vi "Gui_Set_Lamp_Refs.vi"(8 "error in (no error)":errorcluster, 9 "Path":path, 10 "EXPERIMENT Inputs":T1={"Setup"="", "Date"="", "User Name"="", "Comment"="", "Experiment Procedures"=[], "Chemical Source"="", "Sample Components"=[], "Species"=[], "Laser 1"={"Used"=TRUE, "Name"="Spectroscopy", "Wavelength"=1000.0, "Energy"=25.0}, "Laser 2"={"Used"=TRUE, "Name"="Spectroscopy", "Wavelength"=1000.0, "Energy"=25.0}, "Laser 3"={"Used"=TRUE, "Name"="Spectroscopy", "Wavelength"=1000.0, "Energy"=25.0}, "Laser 4"={"Used"=TRUE, "Name"="Spectroscopy", "Wavelength"=1000.0, "Energy"=25.0}, "Laser 5"={"Used"=TRUE, "Name"="Spectroscopy", "Wavelength"=1000.0, "Energy"=25.0}, "Lamp 1"={"Used"=TRUE, "Name"="Spectroscopy", "Wavelength"=1000.0, "Attenuation"=25.0}, "Lamp 2"={"Used"=TRUE, "Name"="Spectroscopy", "Wavelength"=1000.0, "Attenuation"=25.0}, "Gas 1"={"Used"=TRUE, "Name"="Spectroscopy", "Pressure"=1000.0}, "Gas 2"={"Used"=TRUE, "Name"="Spectroscopy", "Pressure"=1000.0}, "Gas 3"={"Used"=TRUE, "Name"="Spectroscopy", "Pressure"=1000.0}, "Gas 4"={"Used"=TRUE, "Name"="Spectroscopy", "Pressure"=1000.0}, "Gas 5"={"Used"=TRUE, "Name"="Spectroscopy", "Pressure"=1000.0}}, 11 "Lamp Refs":refnum<vi>[](array[refnum])) -> (0 "error out":errorcluster caption="sortie d'erreur", 3 "Lamp Refs out":refnum<vi>[](array[refnum]))   [LabVIEW 2017]
uses:
  controls/EXPERIMENT_Inputs.ctl
  controls/LASER_Inputs.ctl
  controls/LAMP_Inputs.ctl
  controls/GAS_Inputs.ctl
panel:
  # "Lasers"
  # "nm"
  # "mJ"
  # "Lamps"
  # "nm"
  # "dB"
  # "Gas"
  # "bar"
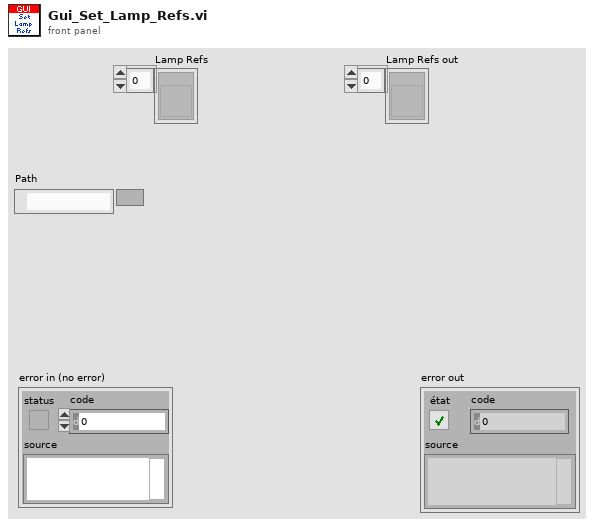
[diagram p1: front panel]
types:
  T1 = typedef "EXPERIMENT_Inputs.ctl" = cluster{"Setup":string, "Date":string, "User Name":string, "Comment":string, "Experiment Procedures":string[], "Chemical Source":string, "Sample Components":string[], "Species":string[], "Laser 1":T2, "Laser 2":T2, "Laser 3":T2, "Laser 4":T2, "Laser 5":T2, "Lamp 1":T3, "Lamp 2":T3, "Gas 1":T4, "Gas 2":T4, "Gas 3":T4, "Gas 4":T4, "Gas 5":T4}
  T2 = typedef "LASER_Inputs.ctl" = cluster{"Used":bool, "Name":string, "Wavelength":dbl, "Energy":dbl}
  T3 = typedef "LAMP_Inputs.ctl" = cluster{"Used":bool, "Name":string, "Wavelength":dbl, "Attenuation":dbl}
  T4 = typedef "GAS_Inputs.ctl" = cluster{"Used":bool, "Name":string, "Pressure":dbl}
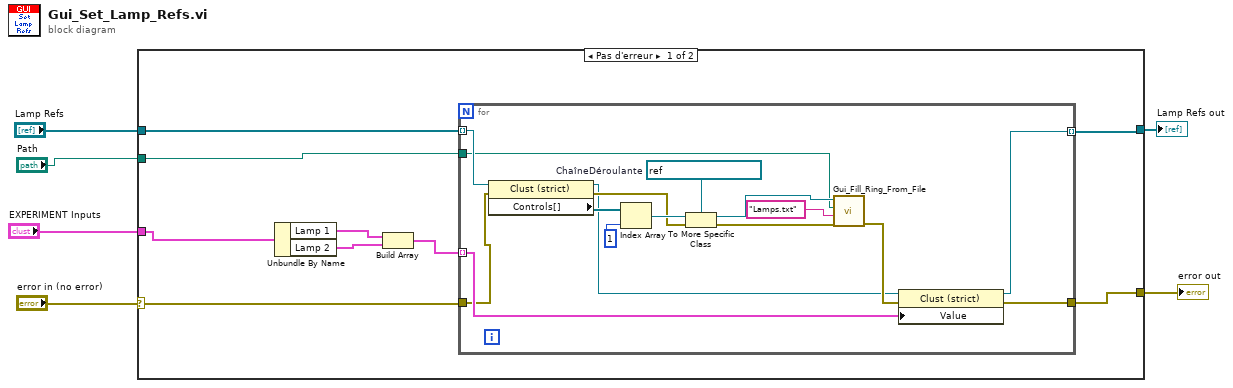
[diagram p0: block diagram]
diagram:
  n1 = case shown="Pas d'erreur" "error in (no error)" {
    selector: "error in (no error)" -> [w15 w33]
    tunnel: [w10 w33] -> w6
    tunnel: [w11 w32] -> w2
    tunnel: "Path" -> [w9 _]
    tunnel: "Lamp Refs" -> [w8 w32]
    tunnel: "EXPERIMENT Inputs" -> [w7 _]
    frame No Error {
      n2 = Unbundle By Name(w7) -> ("Lamp 1"=w13:T3, "Lamp 2"=w14:T3)
      n3 = Build Array(w13, w14) -> (w12:T3[])
      n4 = for {
        tunnel: w12 -> [w31] mode=indexing
        tunnel: w8 -> [w22] mode=indexing
        tunnel: [w30] -> w11 mode=indexing
        tunnel: w15 -> [w21]
        tunnel: [w29] -> w10
        tunnel: w9 -> [w19]
        w23 = refnum<vi> refnum  # ChaîneDéroulante
        n5 = property class="Clust (strict)"(reference=w22, error in=w21) -> (reference out=w17:refnum<vi>, error out=w20:errorcluster, "Controls[]"=w27:refnum<vi>[])
        n6 = Index Array(array=w27, index=1 ("indice")) -> (element=w25:refnum<vi>)
        n7 = To More Specific Class(target class=w23, reference=w25, error in=w20) -> (specific class reference=w24:refnum<vi>, error out=w16:errorcluster)
        n8 = call "Gui_Fill_Ring_From_File.vi"("error in (no error)"=w16, "Resource Name"="Lamps.txt", "Resource Path"=w19, "Refnum ChneDér"=w24) -> ("error out"=w18:errorcluster)  [unwired: 4 in, 3 out]
        n9 = property class="Clust (strict)"(reference=w17, error in=w18, "Value"=w31) -> (reference out=w30:refnum<vi>, error out=w29:errorcluster)
      }
    }
    frame Error {
    }
  }
  "error out" <- w6
  "Lamp Refs out" <- w2
